vi "Anritsu_MT8852B_YYLL_Inquiry.vi"(8 "error in (no error)":errorcluster, 11 "VISA resource in":refnum<visa-resource-name>="GPIB0::27::INSTR") -> (0 "error out":errorcluster, 2 "MAC":string, 3 "VISA resource out":refnum<visa-resource-name>)   [LabVIEW 2017]
panel:
  out "Show":bool
  out "read INQRSP":string
  # "INQUIRY"
  # "MT8852B"
  # "Anritsu"
  # "YYLL"
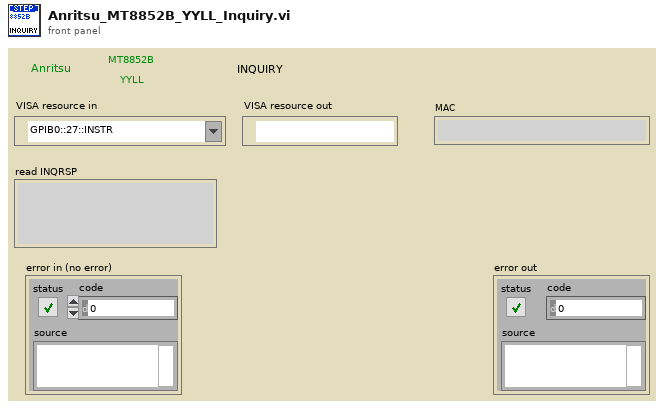
[diagram p1: front panel]
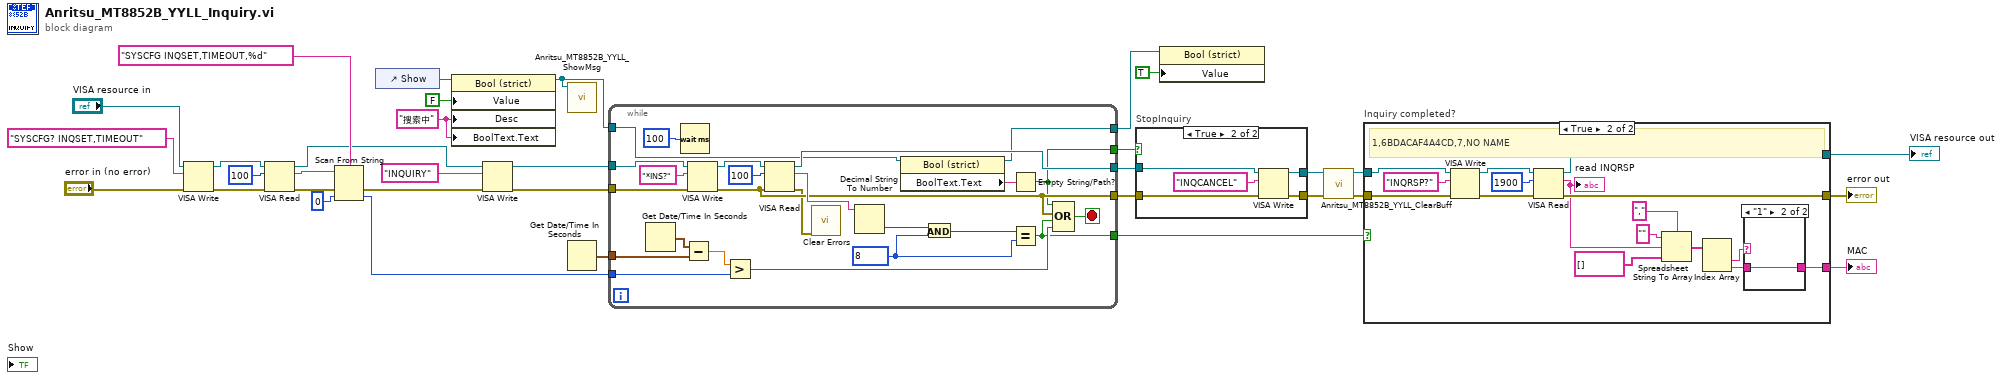
[diagram p0: block diagram]
diagram:
  w6 = "搜索中" ("String")
  n1 = VISA Write(VISA resource name="VISA resource in", write buffer="SYSCFG? INQSET,TIMEOUT", error in (no error)="error in (no error)") -> (VISA resource name out=w32:refnum<visa-resource-name>, error out=w33:errorcluster)  [unwired: 1 out]
  n2 = VISA Read(VISA resource name=w32, byte count=u32 100 ("byte count (0)"), error in (no error)=w33) -> (VISA resource name out=w26:refnum<visa-resource-name>, read buffer=w29:string, error out=w28:errorcluster)  [unwired: 1 out]
  n3 = Scan From String(format string="SYSCFG INQSET,TIMEOUT,%d", input string=w29, error in=w28, default 1=u32 0 ("default value 1")) -> (error out=w27:errorcluster, output 1=w21:u32)  [unwired: 1 in, 2 out]
  n4 = control-ref of="Show"() -> (w13:refnum<vi>)
  n5 = property on="Property Node" class="Bool (strict)"(reference=w13, "Value"=FALSE, "Desc"=w6, "BoolText.Text"=w6) -> (reference out=w9:refnum<vi>)  [unwired: 1 in, 1 out]
  n6 = VISA Write(VISA resource name=w26, write buffer="INQUIRY", error in (no error)=w27) -> (VISA resource name out=w17:refnum<visa-resource-name>, error out=w16:errorcluster)  [unwired: 1 out]
  n7 = call "Anritsu_MT8852B_YYLL_ShowMsg.vi"("reference out"=w9) -> ()  [unwired: 11 in]
  n8 = Get Date/Time In Seconds() -> (seconds since 1Jan1904=w18:timestamp)
  n9 = while {
    tunnel: w17 -> [w47]
    tunnel: [w45] -> w3
    tunnel: [w40] -> w2
    tunnel: w18 -> [w54]
    tunnel: w16 -> [w44]
    tunnel: w21 -> [w43]
    tunnel: [w41] -> w15
    tunnel: [w38] -> w10
    tunnel: w9 -> [w37]
    tunnel: [w35] -> w5
    stop <- w56 stop-if-true
    w57 = 8 ("y")
    n10 = Get Date/Time In Seconds() -> (seconds since 1Jan1904=w55:timestamp)
    n11 = Wait (ms)(milliseconds to wait=u32 100) -> ()  [unwired: 1 out]
    n12 = Subtract(x=w55, y=w54) -> (x-y=w53:dbl)
    n13 = VISA Write(VISA resource name=w47, write buffer="*INS?" ("write buffer (\"\")"), error in (no error)=w44) -> (VISA resource name out=w49:refnum<visa-resource-name>, error out=w40:errorcluster)  [unwired: 1 out]
    n14 = Greater?(x=w53, y=w43) -> (0:w52:bool)
    n15 = VISA Read(VISA resource name=w49, byte count=u32 100 ("byte count (0)"), error in (no error)=w40) -> (VISA resource name out=w45:refnum<visa-resource-name>, read buffer=w51:string, error out=w39:errorcluster)  [unwired: 1 out]
    n16 = call <vilib>:"Clear Errors.vi"("error in (no error)"=w39) -> ()  [unwired: 5 in, 2 out]
    n17 = Decimal String To Number(string=w51) -> (number=w46:i32)  [unwired: 2 in, 1 out]
    n18 = property on="Property Node" class="Bool (strict)"(reference=w37) -> (reference out=w38:refnum<vi>, "BoolText.Text"=w36:string)  [unwired: 1 in, 1 out]
    n19 = And(x=w46, y=w57) -> (x .and. y?=w58:i32)
    n20 = Empty String/Path?(string/path=w36) -> (empty?=w35:bool)
    n21 = Equal?(x=w58, y=w57) -> (x = y?=w41:bool)
    n22 = Compound Arithmetic op=OR(w35, w40, w41, w52) -> (w56:bool)
  }
  n23 = case "StopInquiry" shown="True" w5 {
    tunnel: [w60 w65] -> w4
    tunnel: w3 -> [w60 w64]
    tunnel: w2 -> [w59 w62]
    tunnel: [w59 w61] -> w1
    frame False {
    }
    frame True {
      n24 = VISA Write(VISA resource name=w64, write buffer="INQCANCEL", error in (no error)=w62) -> (VISA resource name out=w65:refnum<visa-resource-name>, error out=w61:errorcluster)  [unwired: 1 out]
    }
  }
  n25 = property on="Property Node" class="Bool (strict)"(reference=w10, "Value"=TRUE) -> ()  [unwired: 1 in, 2 out]
  n26 = call "Anritsu_MT8852B_YYLL_ClearBuff.vi"("error IO"=w1, "VISA resource name"=w4) -> ("error IO 2"=w8:errorcluster, "VISA resource name 2"=w7:refnum<visa-resource-name>)  [unwired: 7 in, 1 out]
  n27 = case "Inquiry completed?" shown="True" w15 {
    tunnel: w7 -> [w66 w79]
    tunnel: w8 -> [w67 w78]
    tunnel: [w67 w76] -> w23
    tunnel: [_ w68] -> w24
    tunnel: [w66 w77] -> w22
    frame False {
    }
    frame True {
      # "1,6BDACAF4A4CD,7,NO NAME"
      n28 = VISA Write(VISA resource name=w79, write buffer="INQRSP?" ("write buffer (\"\")"), error in (no error)=w78) -> (VISA resource name out=w82:refnum<visa-resource-name>, error out=w81:errorcluster)  [unwired: 1 out]
      n29 = VISA Read(VISA resource name=w82, byte count=u32 1900 ("byte count (0)"), error in (no error)=w81) -> (VISA resource name out=w77:refnum<visa-resource-name>, read buffer=w75:string, error out=w76:errorcluster)  [unwired: 1 out]
      "read INQRSP" <- w75
      n30 = Spreadsheet String To Array(delimiter (Tab)=",", format string="", spreadsheet string=w75, array type (2D Dbl)=string[] []) -> (array=w72:string[])
      n31 = Index Array(array=w72) -> (element #1=w70:string, element #2=w69:string)  [unwired: 2 in]
      n32 = case shown="\"1\"" w70 {
        tunnel: [_ w84] -> w68
        tunnel: w69 -> [_ w84]
        frame "False", Default {
        }
        frame "1" {
        }
      }
    }
  }
  "MAC" <- w24
  "error out" <- w23
  "VISA resource out" <- w22
